vi "YAFFooter_ClassCast.vi"(11 "YAFFooter:YAFFooter in":refnum<class>) -> (3 "YAFFooter:YAFFooter out":refnum<class "YAFFooter.lvclass">)   [LabVIEW 2021, in "YAFFooter.lvlib" / "YAFFooter.lvclass"]
uses:
  YAFFooter.lvclass
  YAFFooter.lvclass/YAFFooter.ctl
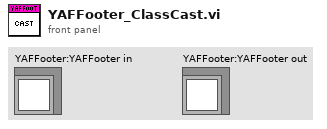
[diagram p1: front panel]
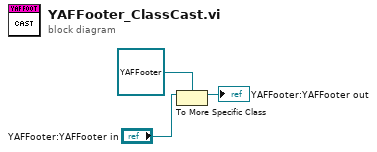
[diagram p0: block diagram]
diagram:
  n1 = To More Specific Class(target class=refnum<class "YAFFooter.lvclass"> refnum ("reference in"), reference="YAFFooter:YAFFooter in") -> (specific class reference=→"YAFFooter:YAFFooter out":refnum<class "YAFFooter.lvclass">)  [unwired: 1 in, 1 out]
